vi "Get Automatic Focus Mode.vi"(8 "error in (no error)":errorcluster, 11 "Stream in":refnum<class "Stream.lvclass">) -> (0 "error out":errorcluster, 1 "Is Supported":bool, 2 "Automatic Parameter Mode":T1, 3 "Stream (Duplicate)":refnum<class "Stream.lvclass">)   [LabVIEW 2020, in "capture.lvlib" / "Stream.lvclass"]
uses:
  Stream.lvclass
  Camera Automatic Parameter Mode.ctl
  Camera Automatic Parameters.ctl
  Stream.lvclass/Stream.ctl
  common/Module Path.vi
  <vilib>/Utility/error.llb/Error Cluster From Error Code.vi
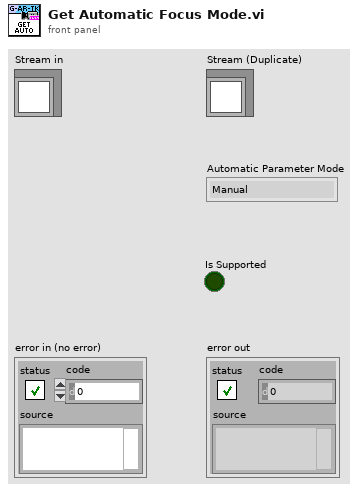
[diagram p1: front panel]
types:
  T1 = typedef "capture.lvlib/Stream.lvclass/Camera Automatic Parameter Mode.ctl" = enum16{"Manual", "Automatic"}
  T2 = typedef "capture.lvlib/Stream.lvclass/Camera Automatic Parameters.ctl" = enum16{"AUTO_EXPOSURE", "AUTO_FOCUS", "AUTO_WHITE_BALANCE", "AUTO_GAIN"}
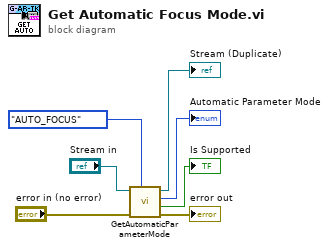
[diagram p0: block diagram]
diagram:
  n1 = call "GetAutomaticParameterMode.vi"("Auto Parameter"=Camera_Automatic_Parameters."AUTO_FOCUS", "error in (no error)"="error in (no error)", "Stream in"="Stream in") -> ("error out"=→"error out":errorcluster, "Is Supported"=→"Is Supported":bool, "Automatic Parameter Mode"=→"Automatic Parameter Mode":T1, "Stream (Duplicate)"=→"Stream (Duplicate)":refnum<class "Stream.lvclass">)  [unwired: 5 in]
